vi "Process-message.vi"(8 "error in (no error)":errorcluster, 10 "Message":refnum<class "Message.lvclass">, 11 "ModComm in":T1) -> (0 "error out":errorcluster, 3 "ModComm out":T1)   [LabVIEW 2013, in "SLMServer.lvlib" / "SLMServer.lvclass"]
uses:
  SLMServer.lvclass
  Object-reference.ctl
  SA-SLMAPI/Sources/Message.lvclass
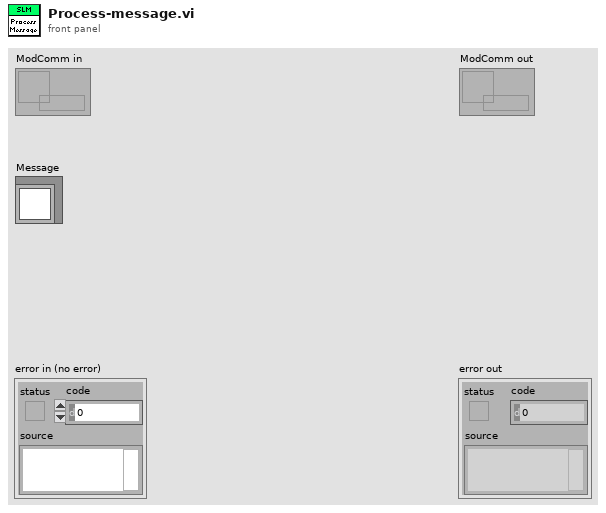
[diagram p1: front panel]
types:
  T1 = typedef "SLMServer.lvlib/SLMServer.lvclass/Object-reference.ctl" = refnum<data-value>
  T2 = typedef "SLMServer.lvlib/SLMServer.lvclass/Server-messages.ctl" = enum16{"Heartbeat", "Error", "Start client", "Client stopped", "Get clients"}
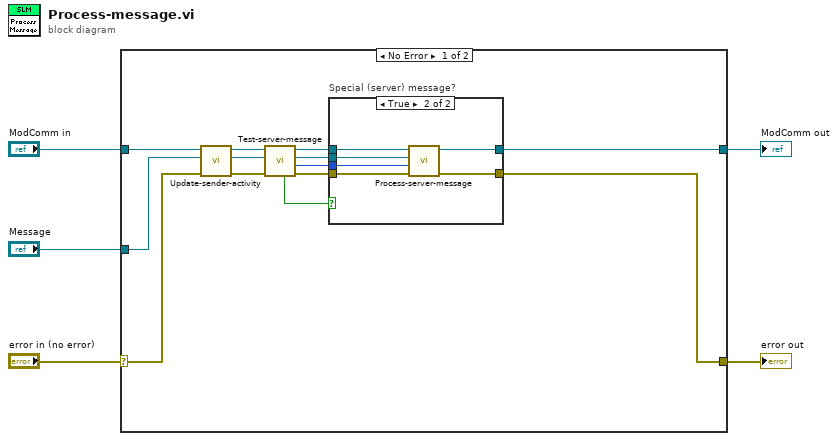
[diagram p0: block diagram]
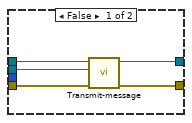
[diagram p2: hidden frame]
diagram:
  n1 = case shown="No Error" "error in (no error)" {
    selector: "error in (no error)" -> [w7 w31]
    tunnel: [w14 w31] -> w4
    tunnel: [w15 w30] -> w2
    tunnel: "ModComm in" -> [w11 w30]
    tunnel: "Message" -> [w6 _]
    frame No Error {
      n2 = call "Update-sender-activity.vi"("error in (no error)"=w7, "Message"=w6, "ModComm in"=w11) -> ("error out"=w8:errorcluster, "Message dup"=w9:refnum<class "Message.lvclass">, "ModComm out"=w10:T1)  [unwired: 6 in]
      n3 = call "Test-server-message.vi"("error in (no error)"=w8, "Message"=w9, "ModComm in"=w10) -> ("error out"=w16:errorcluster, "Server message type"=w12:T2, "Message dup"=w17:refnum<class "Message.lvclass">, "ModComm out"=w18:T1, "Server message?"=w13:bool)  [unwired: 4 in]
      n4 = case "Special (server) message?" shown="True" w13 {
        tunnel: w18 -> [w23 w28]
        tunnel: w17 -> [w21 w29]
        tunnel: w16 -> [w22 w26]
        tunnel: [w20 w25] -> w14
        tunnel: [w19 w27] -> w15
        tunnel: w12 -> [_ w24]
        frame False {
          n5 = call "Transmit-message.vi"("error in (no error)"=w22, "Message"=w21, "ModComm in"=w23) -> ("error out"=w20:errorcluster, "ModComm out"=w19:T1)  [unwired: 7 in]
        }
        frame True {
          n6 = call "Process-server-message.vi"("error in (no error)"=w26, "Message type"=w24, "Message"=w29, "ModComm in"=w28) -> ("error out"=w25:errorcluster, "ModComm out"=w27:T1)  [unwired: 6 in]
        }
      }
    }
    frame Error {
    }
  }
  "error out" <- w4
  "ModComm out" <- w2
